vi "checkBeginPrepareKickoffAllyPlay.vi"(8 "error in (no error)":errorcluster, 10 "Game":refnum<class "Game.lvclass">, 11 "PrepareKickoffAllyPlay in":refnum<class "PrepareKickoffAllyPlay.lvclass">) -> (0 "error out":errorcluster, 2 "Boolean":bool, 3 "PrepareKickoffAllyPlay out":refnum<class "PrepareKickoffAllyPlay.lvclass">)   [LabVIEW 2018, in "PrepareKickoffAllyPlay.lvclass"]
uses:
  PrepareKickoffAllyPlay.lvclass
  Game_class/Game.lvclass
  Game_class/Game.lvclass/Game.ctl
  Referee_class/Referee.lvclass/Referee.ctl
  Referee_class/command_interpreted.ctl
  Game_class/Read Referee.vi
  Referee_class/Read command_interpreted.vi
  Referee_class/Referee.lvclass
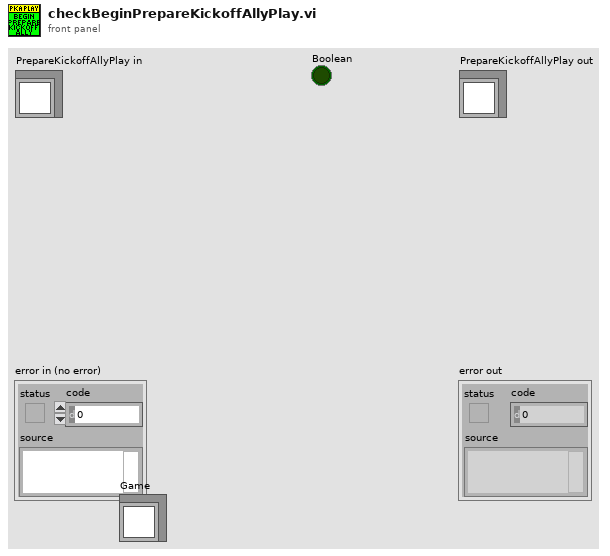
[diagram p1: front panel]
types:
  T1 = typedef "command_interpreted.ctl" = enum16{"Goal Ally", "Goal Enemy", "Ball Placement Enemy", "Ball Placement Ally", "Normal Half Time", "Extra Time  Break", "Extra Half Time", "None", "Post Game", "PKA Normal Start", "Prepare Kickoff Ally", "PKE Normal Start", "Prepare Kickoff Enemy", "Force Start", "Halt", "Timeout", "Prepare Penalty Ally", "Prepare Penalty Enemy", "PPA NormalStart", "PPE Normal Start", "Indirect Free Ally", "Direct Free Enemy", "Direct Free Ally", "Indirect Free Enemy", "Stop"}
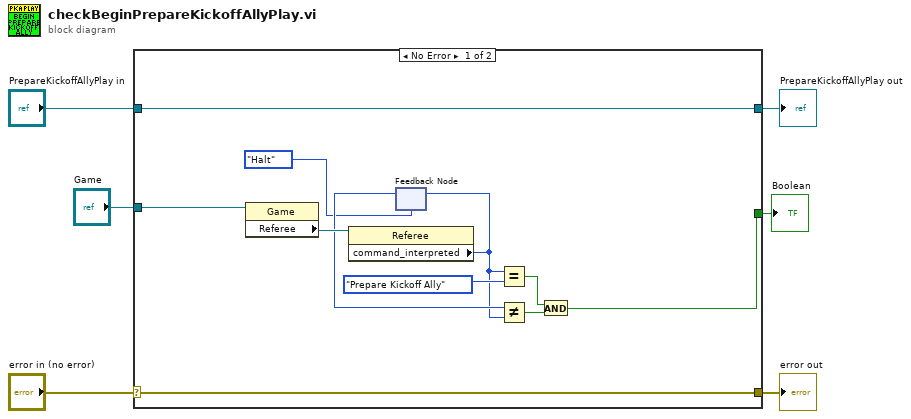
[diagram p0: block diagram]
diagram:
  n1 = case shown="No Error" "error in (no error)" {
    selector: "error in (no error)" -> [w16 w19]
    tunnel: [w16 w19] -> w5
    tunnel: [w17 w18] -> w3
    tunnel: "PrepareKickoffAllyPlay in" -> [w17 w18]
    tunnel: "Game" -> [w9 _]
    tunnel: [w8 _] -> w1
    frame No Error {
      n2 = property class="Game"(reference=w9) -> ("Referee"=w15:refnum<class "Referee.lvclass">)  [unwired: 1 in, 2 out]
      n3 = property class="Referee"(reference=w15) -> ("command_interpreted"=w11:T1)  [unwired: 1 in, 2 out]
      n4 = feedback #1(command_interpreted."Halt" ("command_interpreted")) -> (w12:T1)
      n5 = feedback-in #1(w11) -> ()
      n6 = Equal?(x=w11, y=command_interpreted."Prepare Kickoff Ally" ("command_interpreted")) -> (x = y?=w13:bool)
      n7 = Not Equal?(x=w12, y=w11) -> (x != y?=w10:bool)
      n8 = And(x=w13, y=w10) -> (x .and. y?=w8:bool)
    }
    frame Error {
    }
  }
  "error out" <- w5
  "PrepareKickoffAllyPlay out" <- w3
  "Boolean" <- w1
